vi "Gate Data.vi"(0 "Data In":dbl[](array[numeric]), 1 "Gate Center":u32, 2 "Gate Width":u32) -> (3 "Gated Data Out":dbl[](array[numeric]), 4 "Indeces Used":i32[](array[numeric]), 5 "% population in gate":dbl, 6 "Gate Position (min,max)":dbl[](array[numeric]))   [LabVIEW 2012]
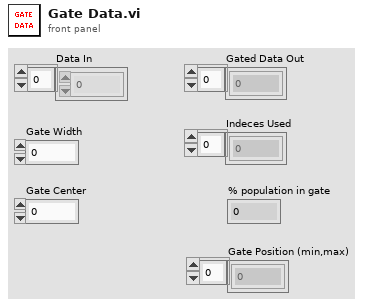
[diagram p1: front panel]
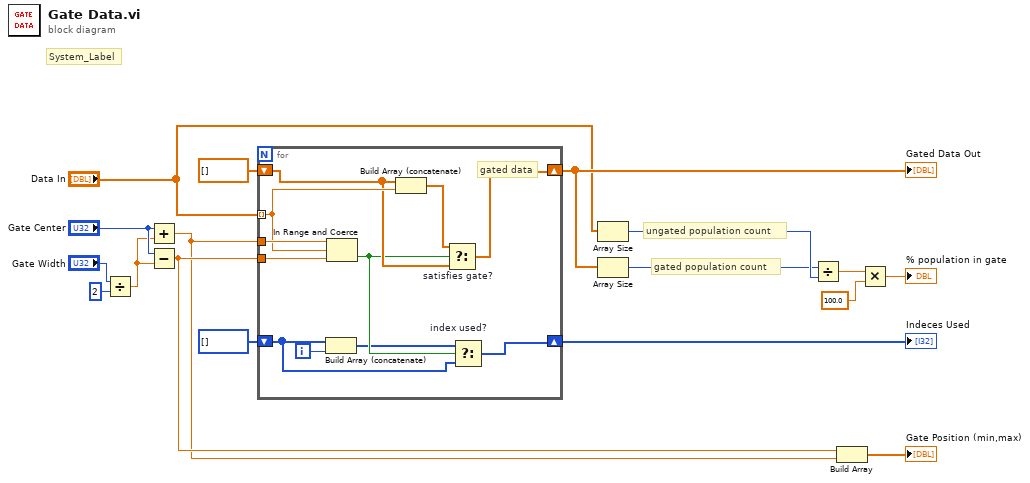
[diagram p0: block diagram]
diagram:
  # "System_Label"
  # "gated population count"
  # "ungated population count"
  n1 = Divide(x="Gate Width", y=u32 2) -> (x/y=w4:dbl)
  n2 = Add(x="Gate Center", y=w4) -> (x+y=w2:dbl)
  n3 = Subtract(x="Gate Center", y=w4) -> (x-y=w3:dbl)
  n4 = for "Gate micron index of intensiy peaks" {
    tunnel: "Data In" -> [w26] mode=indexing
    tunnel: w3 -> [w27]
    tunnel: w2 -> [w28]
    shift-right: [w25] -> w11
    shift-left: dbl[] [] -> [w23]
    shift-right: [w18] -> w8
    shift-left: i32[] [] -> [w19]
    i -> [w21]
    # "gated data"
    n5 = Build Array (concatenate)(w19, w21) -> (w20:i32[])
    n6 = In Range and Coerce(upper limit=w28, x=w26, lower limit=w27) -> (In Range?=w22:bool)  [unwired: 1 out]
    n7 = Build Array (concatenate)(w23, w26) -> (w24:dbl[])
    n8 = Select "satisfies gate?"(t=w24, s=w22, f=w23) -> (s? t:f=w25:dbl[])
    n9 = Select "index used?"(t=w20, s=w22, f=w19) -> (s? t:f=w18:i32[])
  }
  "Gated Data Out" <- w11
  "Indeces Used" <- w8
  n10 = Array Size(array="Data In") -> (size(s)=w13:i32)
  n11 = Array Size(array=w11) -> (size(s)=w12:i32)
  n12 = Divide(x=w12, y=w13) -> (x/y=w14:dbl)
  n13 = Build Array(w3, w2) -> (→"Gate Position (min,max)":dbl[])
  n14 = Multiply(x=w14, y=100.0) -> (x*y=→"% population in gate":dbl)
